vi "Next Step.vi"(8 "error in (no error)":errorcluster, 11 "ControlClassWizard in":refnum<class "QControl Creation Wizard.lvclass">) -> (0 "error out":errorcluster, 1 "Finish Button?":bool, 2 "Finish Script?":bool, 3 "ControlClassWizard out":refnum<class "QControl Creation Wizard.lvclass">)   [LabVIEW 2015, in "QControl Creation Wizard.lvclass"]
doc: "<b> </b> <b> </b>\n©2016 Q Software Innovations, LLC (QSI)\nwritten by Quentin Alldredge\nproduced in LabVIEW 2015\n\nsupport@qsoftwareinnovations.com\nwww.qsoftwareinnovations.com\n\nAll rights reserved.\n\nRedistribution and use in source and binary forms, with or without modification, are permitted provided that the following conditions are met:\n\n * Redistributions of source code must retain the above copyright notice, this list of conditions and the following disclaimer.\n * Redistributions in binary form must reproduce the above copyright notice, this list of conditions and the following disclaimer in the documentation and/or other materials provided with the distribution.\n * Neither the name of Q Software Innovations, LLC. nor the names of its contributors may be used to endorse or promote products derived from this software without specific prior written permission.\n\nTHIS SOFTWARE IS PROVIDED BY THE COPYRIGHT HOLDERS AND CONTRIBUTORS \"AS IS\" AND ANY EXPRESS OR IMPLIED WARRANTIES, INCLUDING, BUT NOT LIMITED TO, THE IMPLIED WARRANTIES OF MERCHANTABILITY AND FITNESS FOR A PARTICULAR PURPOSE ARE DISCLAIMED. IN NO EVENT SHALL THE COPYRIGHT OWNER OR CONTRIBUTORS BE LIABLE FOR ANY DIRECT, INDIRECT, INCIDENTAL, SPECIAL, EXEMPLARY, OR CONSEQUENTIAL DAMAGES (INCLUDING, BUT NOT LIMITED TO, PROCUREMENT OF SUBSTITUTE GOODS OR SERVICES; LOSS OF USE, DATA, OR PROFITS; OR BUSINESS INTERRUPTION) HOWEVER CAUSED AND ON ANY THEORY OF LIABILITY, WHETHER IN CONTRACT, STRICT LIABILITY, OR TORT (INCLUDING NEGLIGENCE OR OTHERWISE) ARISING IN ANY WAY OUT OF THE USE OF THIS SOFTWARE, EVEN IF ADVISED OF THE POSSIBILITY OF SUCH DAMAGE."
uses:
  QControl Creation Wizard.lvclass
  QControl Creation Wizard.lvclass/QControl Creation Wizard.ctl
  QControl Classes/Steps/Steps.lvclass
  QControl Creation Script/QControl Creation.lvclass
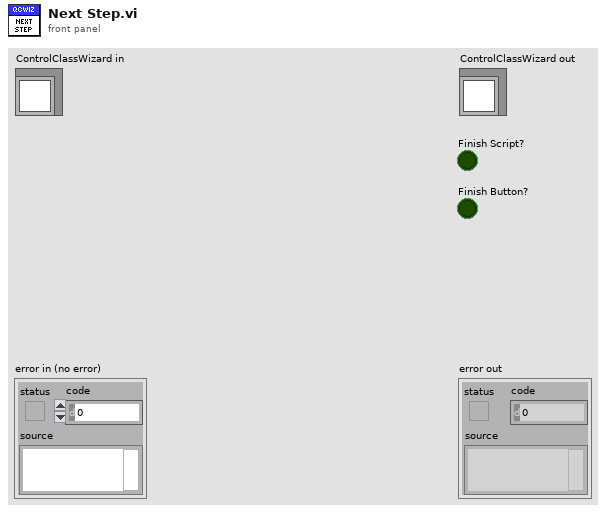
[diagram p1: front panel]
types:
  T1 = enum16{"Don't Add", "To Target", "To Project Item"}
  T2 = typedef "QControl Creation.lvclass/New QControl Information.ctl" = cluster{"QControl Class Name":string, "Localized Name":string, "Description":string, "Parent Class Path":path, "New Class Path":path, "Banner Text":string, "Add to Location":enum16{"Don't Add", "To Target", "To Project Item"}, "Target Ref":refnum<vi>, "ProjectItem Ref":refnum<vi>}
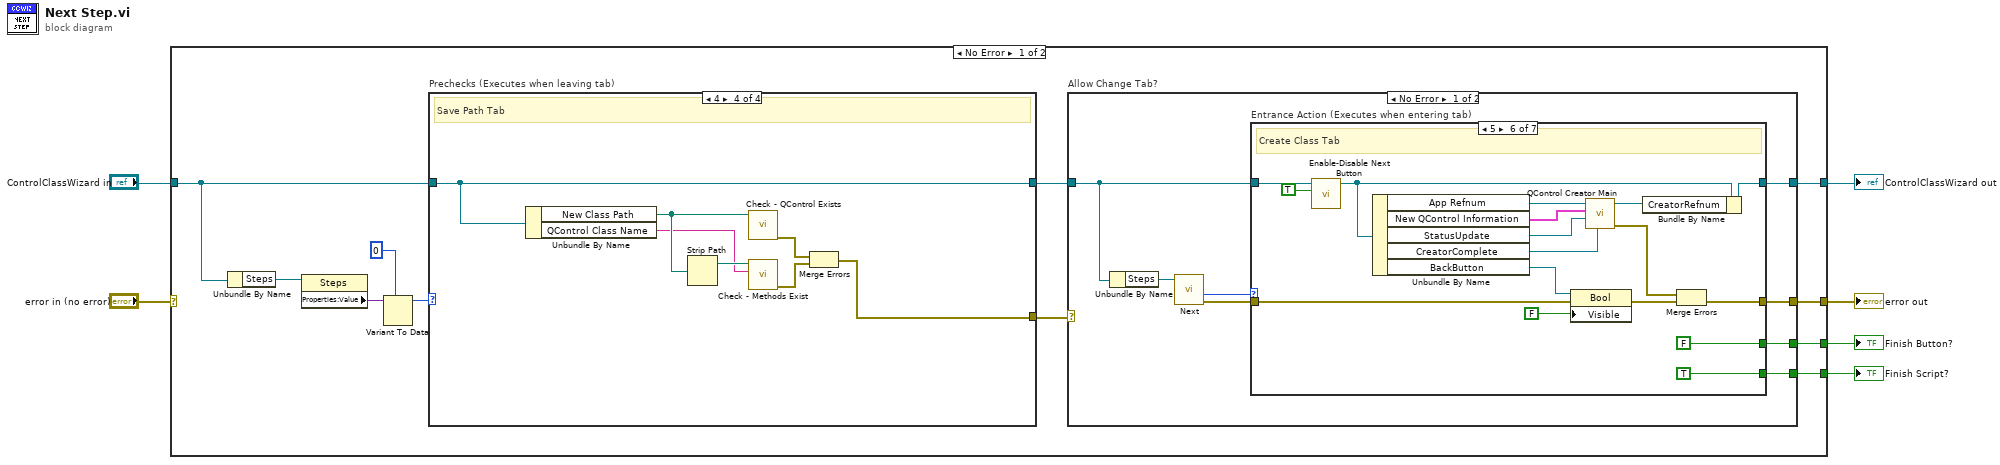
[diagram p0: block diagram]
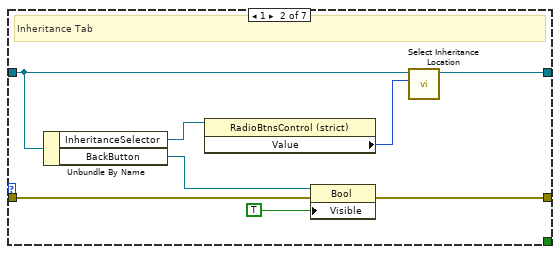
[diagram p3: hidden frame]
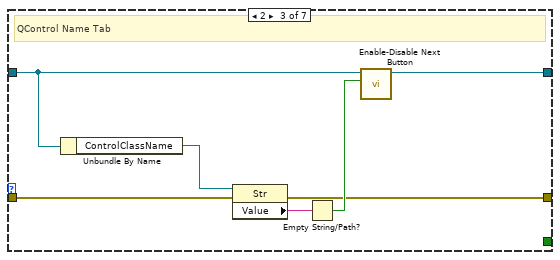
[diagram p4: hidden frame]
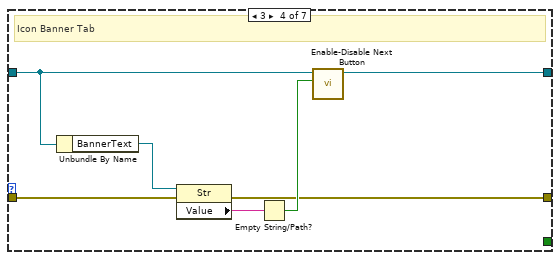
[diagram p5: hidden frame]
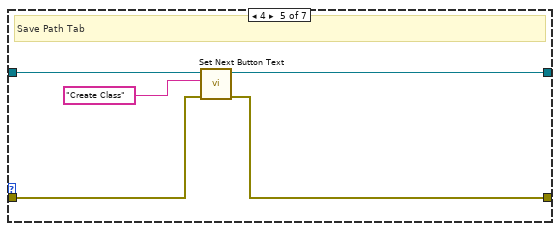
[diagram p6: hidden frame]
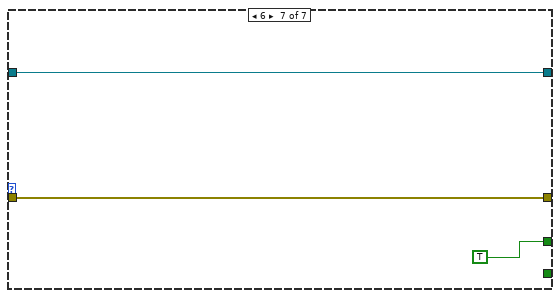
[diagram p7: hidden frame]
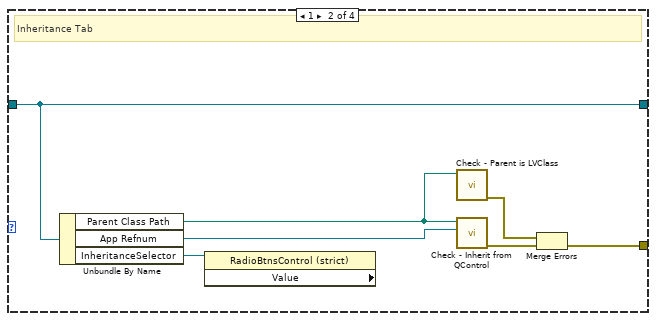
[diagram p10: hidden frame]
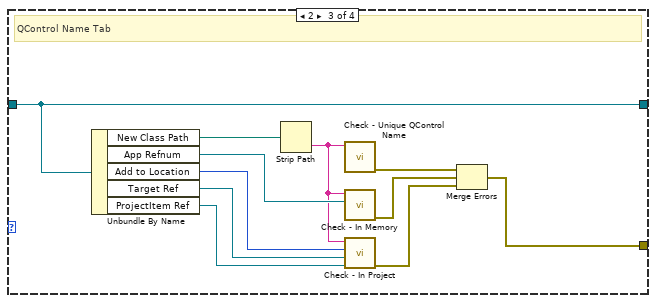
[diagram p11: hidden frame]
diagram:
  n1 = case shown="No Error" "error in (no error)" {
    selector: "error in (no error)" -> [_ w104]
    tunnel: [w15 w104] -> w5
    tunnel: [w16 w103] -> w3
    tunnel: "ControlClassWizard in" -> [w9 w103]
    tunnel: [w17 _] -> w2
    tunnel: [w14 _] -> w1
    frame No Error {
      n2 = Unbundle By Name(w9) -> ("Steps"=w13:refnum<class "Steps.lvclass">)
      n3 = property class="Steps"(reference=w13) -> ("Properties:Value"=w12:variant)  [unwired: 1 in, 2 out]
      n4 = Variant To Data(type=0, Variant=w12) -> (data=w10:i32)  [unwired: 1 in, 1 out]
      n5 = case "Prechecks (Executes when leaving tab)" shown="4" w10 {
        tunnel: w9 -> [w77 w82 w95 w102]
        tunnel: [w77 w82 w95 w102] -> w8
        tunnel: [_ w80 w85 w101] -> w7
        frame Default {
          # "Start Tab, Icon Banner Tab"
        }
        frame 1 {
          # "Inheritance Tab"
          n6 = Unbundle By Name(w82) -> ("Parent Class Path"=w83:path, "App Refnum"=w81:refnum<vi>, "InheritanceSelector"=w84:refnum<vi>)
          n7 = property class="RadioBtnsControl (strict)" props=["Value"](reference=w84) -> ()  [unwired: 1 in, 3 out]
          n8 = call "Check - Parent is LVClass.vi"("Parent Class Path"=w83) -> ("error out"=w78:errorcluster)  [unwired: 10 in]
          n9 = call "Check - Inherit from QControl.vi"("Application in"=w81, "Parent Class Path"=w83) -> ("error out"=w79:errorcluster)  [unwired: 9 in]
          n10 = Merge Errors(w78, w79) -> (w80:errorcluster)
        }
        frame 2 {
          # "QControl Name Tab"
          n11 = Unbundle By Name(w95) -> ("New Class Path"=w94:path, "App Refnum"=w93:refnum<vi>, "Add to Location"=w91:T1, "Target Ref"=w90:refnum<vi>, "ProjectItem Ref"=w89:refnum<vi>)
          n12 = Strip Path(path=w94) -> (name=w92:string)  [unwired: 1 out]
          n13 = call "Check - Unique QControl Name.vi"("QControl Class Name"=w92) -> ("error out"=w88:errorcluster)  [unwired: 10 in]
          n14 = call "Check - In Memory.vi"("Application in"=w93, "QControl Class Name"=w92) -> ("error out"=w87:errorcluster)  [unwired: 9 in]
          n15 = call "Check - In Project.vi"("ProjectItem Ref"=w89, "TargetItem in"=w90, "Add to Location"=w91, "QControl Class Name"=w92) -> ("error out"=w86:errorcluster)  [unwired: 7 in]
          n16 = Merge Errors(w88, w87, w86) -> (w85:errorcluster)
        }
        frame 4 {
          # "Save Path Tab"
          n17 = Unbundle By Name(w102) -> ("New Class Path"=w97:path, "QControl Class Name"=w96:string)
          n18 = Strip Path(path=w97) -> (stripped path=w100:path)  [unwired: 1 out]
          n19 = call "Check - QControl Exists.vi"("New Class Path"=w97) -> ("error out"=w98:errorcluster)  [unwired: 10 in]
          n20 = call "Check - Methods Exist.vi"("QControl Class Name"=w96, "New Class Root Path"=w100) -> ("error out"=w99:errorcluster)  [unwired: 9 in]
          n21 = Merge Errors(w98, w99) -> (w101:errorcluster)
        }
      }
      n22 = case "Allow Change Tab?" shown="No Error" w7 {
        selector: w7 -> [_ w76]
        tunnel: [w23 _] -> w17
        tunnel: [w22 w75] -> w16
        tunnel: [w21 w76] -> w15
        tunnel: [w20 _] -> w14
        tunnel: w8 -> [w19 w75]
        frame No Error {
          n23 = Unbundle By Name(w19) -> ("Steps"=w18:refnum<class "Steps.lvclass">)
          n24 = call "Next.vi"("Steps in"=w18) -> ("error out"=w25:errorcluster, "Step Number"=w24:i32)  [unwired: 7 in, 2 out]
          n25 = case "Entrance Action (Executes when entering tab)" shown="5" w24 {
            tunnel: w25 -> [w27 w35 w42 w49 w54 w71 w73]
            tunnel: [w27 w34 w39 w46 w52 w57 w73] -> w21
            tunnel: [_ _ _ _ _ FALSE TRUE] -> w23
            tunnel: w19 -> [w26 w28 w37 w44 w51 w68 w72]
            tunnel: [w26 w31 w38 w45 w50 w58 w72] -> w22
            tunnel: [_ _ _ _ _ TRUE _] -> w20
            frame Default {
            }
            frame 1 {
              # "Inheritance Tab"
              n26 = Unbundle By Name(w28) -> ("InheritanceSelector"=w29:refnum<vi>, "BackButton"=w30:refnum<vi>)
              n27 = property class="RadioBtnsControl (strict)"(reference=w29) -> ("Value"=w32:enum32{"Tree", "Path"})  [unwired: 1 in, 2 out]
              n28 = property class="Bool"(reference=w30, error in=w35, "Visible"=TRUE) -> (error out=w34:errorcluster)  [unwired: 1 out]
              n29 = call "Select Inheritance Location.vi"("NewVal"=w32, "QControlWizard in"=w28) -> ("QControlWizard (dup)"=w31:refnum<class "QControl Creation Wizard.lvclass">)  [unwired: 8 in, 1 out]
            }
            frame 2 {
              # "QControl Name Tab"
              n30 = Unbundle By Name(w37) -> ("ControlClassName"=w36:refnum<vi>)
              n31 = property class="Str"(reference=w36, error in=w42) -> (error out=w39:errorcluster, "Value"=w41:string)  [unwired: 1 out]
              n32 = Empty String/Path?(string/path=w41) -> (empty?=w40:bool)
              n33 = call "Enable-Disable Next Button.vi"("Disable Next Button?"=w40, "QControlWizard in"=w37) -> ("QControlWizard (dup)"=w38:refnum<class "QControl Creation Wizard.lvclass">)  [unwired: 8 in, 1 out]
            }
            frame 3 {
              # "Icon Banner Tab"
              n34 = Unbundle By Name(w44) -> ("BannerText"=w43:refnum<vi>)
              n35 = property class="Str"(reference=w43, error in=w49) -> (error out=w46:errorcluster, "Value"=w48:string)  [unwired: 1 out]
              n36 = Empty String/Path?(string/path=w48) -> (empty?=w47:bool)
              n37 = call "Enable-Disable Next Button.vi"("Disable Next Button?"=w47, "QControlWizard in"=w44) -> ("QControlWizard (dup)"=w45:refnum<class "QControl Creation Wizard.lvclass">)  [unwired: 8 in, 1 out]
            }
            frame 4 {
              # "Save Path Tab"
              n38 = call "Set Next Button Text.vi"("error in (no error)"=w54, "Text"="Create Class", "QControlWizard in"=w51) -> ("error out"=w52:errorcluster, "QControlWizard (dup)"=w50:refnum<class "QControl Creation Wizard.lvclass">)  [unwired: 7 in]
            }
            frame 5 {
              # "Create Class Tab"
              n39 = call "Enable-Disable Next Button.vi"("Disable Next Button?"=TRUE, "QControlWizard in"=w68) -> ("QControlWizard (dup)"=w59:refnum<class "QControl Creation Wizard.lvclass">)  [unwired: 8 in, 1 out]
              n40 = Unbundle By Name(w59) -> ("App Refnum"=w64:refnum<vi>, "New QControl Information"=w63:T2, "StatusUpdate"=w62:refnum<user-event>, "CreatorComplete"=w61:refnum<user-event>, "BackButton"=w55:refnum<vi>)
              n41 = property class="Bool"(reference=w55, error in=w71, "Visible"=FALSE ("Control:Visible")) -> (error out=w67:errorcluster)  [unwired: 1 out]
              n42 = call "QControl Creator Main.vi"("CreatorComplete"=w61, "StatusUpdate"=w62, "New QControl Information"=w63, "App Refnum"=w64) -> ("error out"=w56:errorcluster, "CreatorRefnum"=w60:refnum<vi>)  [unwired: 6 in]
              n43 = Bundle By Name(cluster=w59, "CreatorRefnum"=w60) -> (w58:refnum<class "QControl Creation Wizard.lvclass">)
              n44 = Merge Errors(w56, w67) -> (w57:errorcluster)
            }
            frame 6 {
            }
          }
        }
        frame Error {
        }
      }
    }
    frame Error {
    }
  }
  "error out" <- w5
  "ControlClassWizard out" <- w3
  "Finish Button?" <- w2
  "Finish Script?" <- w1
